vi "SIM921 Delete Curve.vi"(8 "Error In":errorcluster, 9 "Curve #":i32=1, 10 "Slot":T1(ring), 11 "VISA resource name":refnum<visa-resource-name>) -> (0 "Error Out":errorcluster, 3 "VISA resource name":refnum<visa-resource-name>)   [LabVIEW 2020]
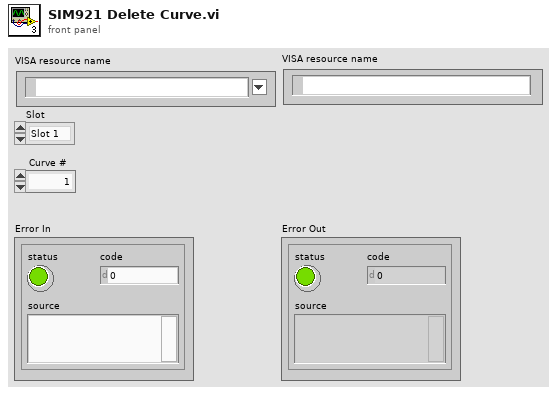
[diagram p1: front panel]
types:
  T1 = enum32{"Slot 1", "Slot 2", "Slot 3", "Slot 4", "Slot 5", "Slot 6", "Slot 7", "Slot 8"}
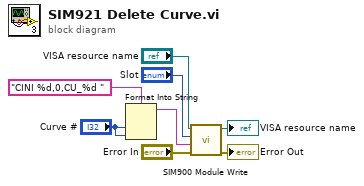
[diagram p0: block diagram]
diagram:
  n1 = Format Into String(format string="CINI %d,0,CU_%d ", "Curve #", "Curve #") -> (resulting string=w3:string)  [unwired: 2 in, 1 out]
  n2 = call "SIM900 Module Write.vi"("Error In"="Error In", "Query"=w3, "Slot"="Slot", "VISA Resource Name"="VISA resource name") -> ("Error Out"=→"Error Out":errorcluster, "dup VISA Session"=→"VISA resource name":refnum<visa-resource-name>)  [unwired: 6 in]
